vi "_Main_05_by_runs.vi"() -> ()   [LabVIEW 2017]
panel:
  out "Log N":u32
  out "Temp, C":dbl
  out "Temp_sp, C":dbl
  out "Temp_gsp, C":dbl
  in  "Start":bool
  in  "SendPeriod, ms":dbl=20.0 min=10.0 max=10000.0
  in  "Graph every, cycle":dbl=1.0 min=1.0 max=100.0
  out "Frame In Run Done":u32
  out "Now is Run #":u32
  out "Global Frame Done":u32
  in  "Frames In Run":u32=180
  in  "Exposition, s":dbl=5.0 min=0.1 max=10.0
  out "Last TrigTimer, s":dbl format="%#.3g"
  in  "LOG file":path=path "F:/_OneDrive/YandexDisk/YandexDisk/Компьютер MAINHOMEPC/OneDrive - Personal/_RF/_Проекты/Термоконтроллер/programming/LabView Side/Null_Log.txt"
  out "Flags":T1
  out "Red LED":bool
  out "Green LED":bool
  in  "Speed, K/min":dbl=5.0 min=0.1 max=10.0
  in  "Target, K":dbl=295.0 min=195.0 max=395.0
  in  "Ramp":bool
  out "Power LOG":cluster{dbl[], dbl[]}(graph)
  in  "Set temp":dbl=195.0 min=195.0 max=395.0
  in  "Setpoint":bool
  out "TrigTimer, s":dbl format="%#_3g"
  out "Vout, V":dbl format="%#.3g"
  out "Vin, V":dbl format="%#.4g"
  out "Temp, K":dbl
  out "Temp_sp, K":dbl
  out "Temp_gsp, K":dbl
  out "Temp LOG":cluster{dbl[], dbl[]}(graph)
  out "Bytes at Port":u32
  out "RecTry":i32
  in  "Stop Button":bool
  in  "COM port":refnum<visa-resource-name>
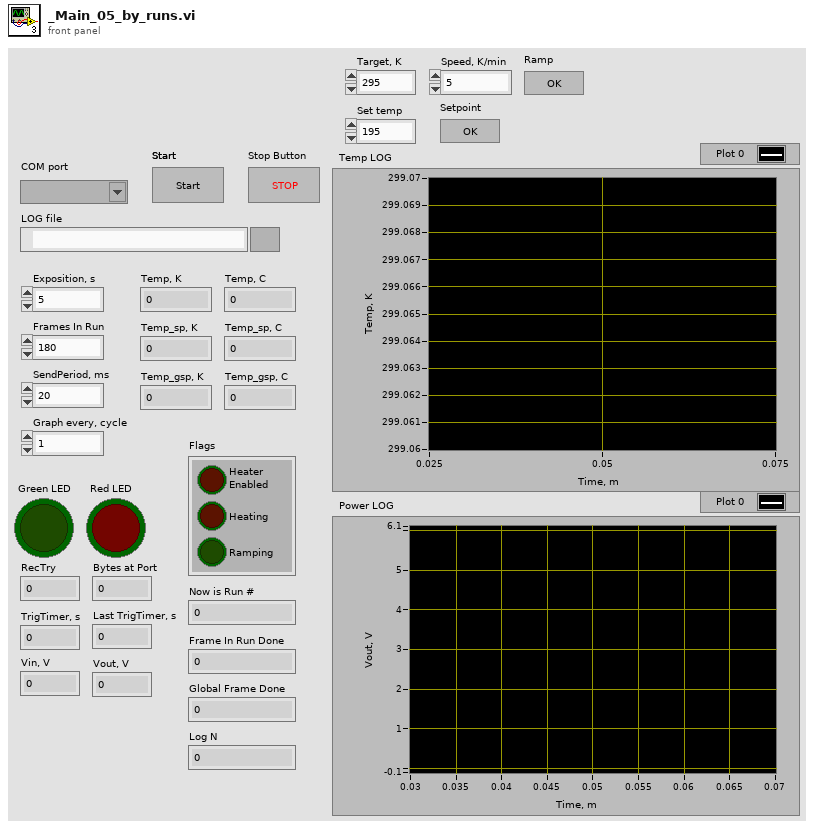
[diagram p1: front panel]
types:
  T1 = cluster{"Heater\nEnabled":bool, "Heating":bool, "Ramping":bool}
  T2 = cluster{i32, i32, u32, "Green LED":bool, "TrigTimer, s":dbl}
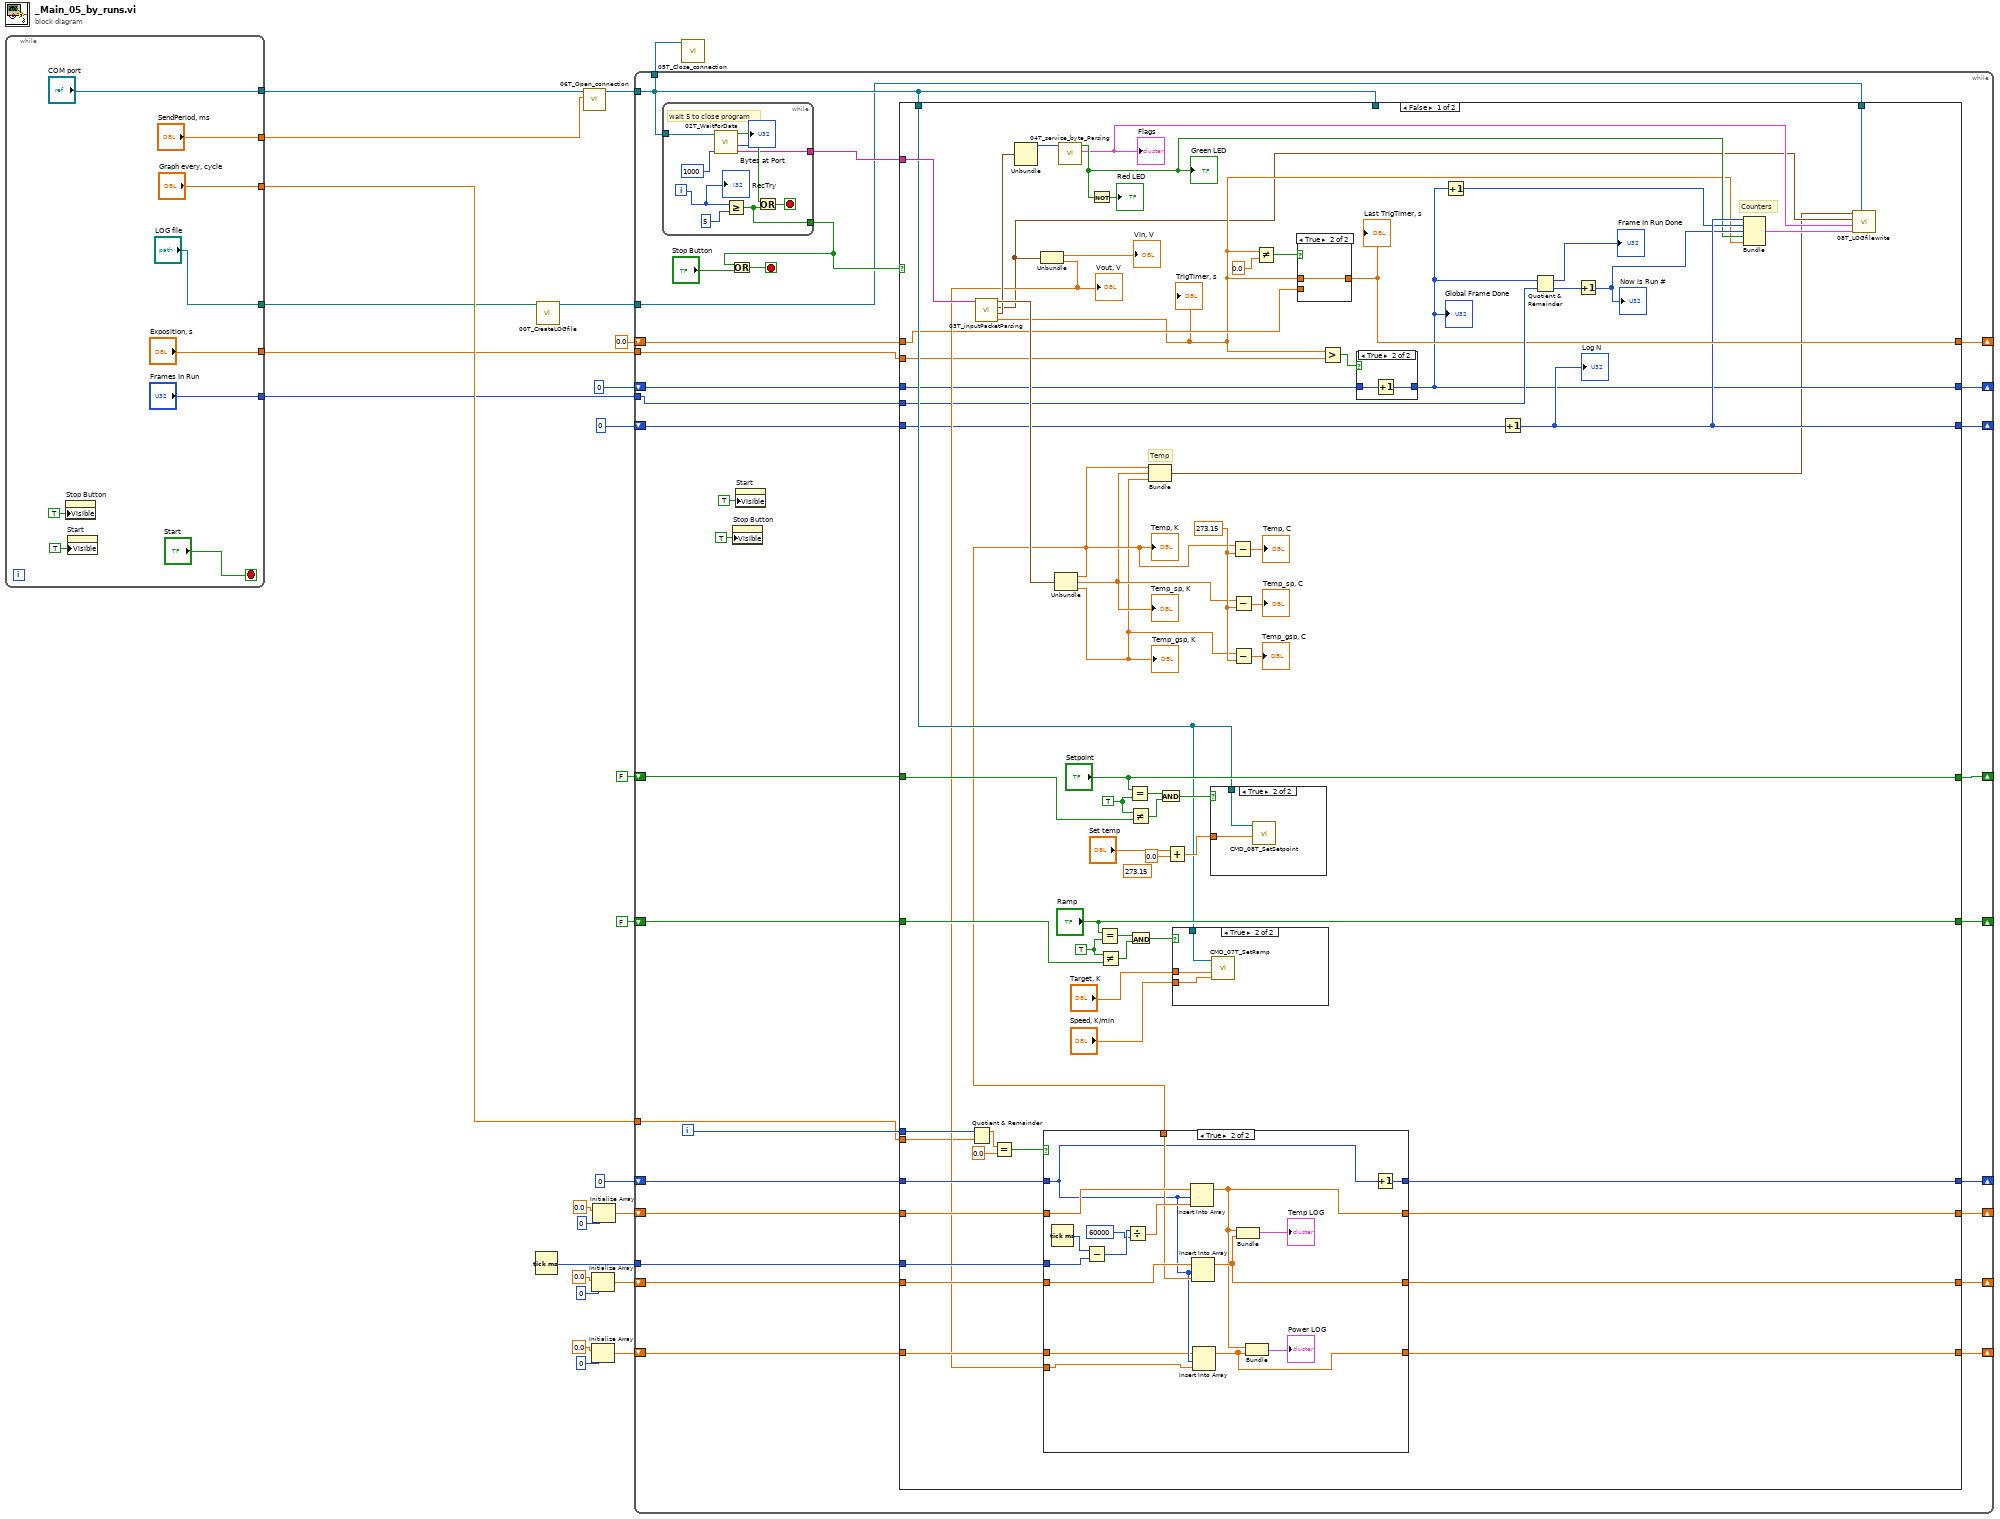
[diagram p0: block diagram]
diagram:
  n1 = while {
    tunnel: ["COM port"] -> w6
    tunnel: ["SendPeriod, ms"] -> w5
    tunnel: ["Graph every, cycle"] -> w4
    tunnel: ["LOG file"] -> w3
    tunnel: ["Frames In Run"] -> w2
    tunnel: ["Exposition, s"] -> w1
    stop <- "Start" stop-if-true
    n2 = property on="Stop Button" class="Bool"("Visible"=TRUE) -> ()  [unwired: 2 in, 2 out]
    n3 = property on="Start" class="Bool"("Visible"=TRUE) -> ()  [unwired: 2 in, 2 out]
  }
  n4 = Tick Count (ms)() -> (millisecond timer value=w21:u32)
  n5 = call "00T_CreateLOGfile.vi"("LOG file"=w3) -> ("refnum out"=w7:refnum<file>)  [unwired: 10 in]
  n6 = call "06T_Open_connection.vi"("Period, ms"=w5, "COM port"=w6) -> ("VISA"=w11:refnum<visa-resource-name>)  [unwired: 9 in]
  n7 = Initialize Array(0.0 ("element"), 0 ("dimension size")) -> (w18:dbl[])
  n8 = Initialize Array(0.0 ("element"), 0 ("dimension size")) -> (w14:dbl[])
  n9 = Initialize Array(0.0 ("element"), 0 ("dimension size")) -> (w22:dbl[])
  n10 = while {
    tunnel: w11 -> [w51]
    tunnel: [w51] -> w12
    shift-right: [w60] -> _
    shift-left: 0 -> [w61]
    tunnel: w21 -> [w58]
    shift-right: [w56] -> _
    shift-left: w22 -> [w59]
    shift-right: [w55] -> _
    shift-left: w18 -> [w57]
    shift-right: [w53] -> _
    shift-left: FALSE ("OK Button") -> [w52]
    shift-right: [w49] -> _
    shift-left: w14 -> [w50]
    shift-right: [w48] -> _
    shift-left: FALSE ("Ramp") -> [w47]
    shift-right: [w46] -> _
    shift-left: 0.0 ("TrigTimer, s") -> [w45]
    shift-right: [w43] -> _
    shift-left: 0 -> [w44]
    shift-right: [w41] -> _
    shift-left: 0 -> [w42]
    tunnel: w7 -> [w40]
    tunnel: w4 -> [w39]
    tunnel: w2 -> [w38]
    tunnel: w1 -> [w37]
    i -> [w62]
    stop <- w65 stop-if-true
    n11 = while {
      tunnel: w51 -> [w174]
      tunnel: [w177] -> w64
      tunnel: [w178] -> w63
      i -> [w176]
      stop <- w180 stop-if-true
      # "wait 5 to close program"
      n12 = call "02T_WaitForData.vi"("WaitTimeoutMS"=u32 1000, "VISA"=w174) -> ("Buffer"=w178:string, "Bytes at Port"=→"Bytes at Port":u32, "Data Recived"=w179:bool)  [unwired: 7 in]
      n13 = Greater Or Equal?(x=w176, y=5) -> (x >= y?=w177:bool)
      n14 = Or(x=w179, y=w177) -> (x .or. y?=w180:bool)
      "RecTry" <- w176
    }
    n15 = Or(x=w64, y="Stop Button") -> (x .or. y?=w65:bool)
    n16 = property on="Stop Button" class="Bool"("Visible"=TRUE) -> ()  [unwired: 2 in, 2 out]
    n17 = property on="Start" class="Bool"("Visible"=TRUE) -> ()  [unwired: 2 in, 2 out]
    n18 = case shown="False" w64 {
      tunnel: w63 -> [w125 _]
      tunnel: w62 -> [w131 _]
      tunnel: w51 -> [_ _]
      tunnel: w61 -> [w129 w173]
      tunnel: [w128 w173] -> w60
      tunnel: w59 -> [w121 w172]
      tunnel: w58 -> [w127 _]
      tunnel: w57 -> [w120 w171]
      tunnel: [w126 w172] -> w56
      tunnel: [w113 w171] -> w55
      tunnel: ["Setpoint" w170] -> w53
      tunnel: w52 -> [w117 w170]
      tunnel: w51 -> [w101 _]
      tunnel: w50 -> [w109 w169]
      tunnel: [w108 w169] -> w49
      tunnel: ["Ramp" w168] -> w48
      tunnel: w47 -> [w103 w168]
      tunnel: [w85 w167] -> w46
      tunnel: w45 -> [w93 w167]
      tunnel: w37 -> [w86 _]
      tunnel: w44 -> [w91 w166]
      tunnel: [w78 w166] -> w43
      tunnel: w38 -> [w90 _]
      tunnel: w39 -> [w87 _]
      tunnel: w42 -> [w80 w165]
      tunnel: [w79 w165] -> w41
      tunnel: w40 -> [w66 _]
      frame False {
        w81 = 273.15
        w104 = TRUE ("y")
        (unwired) 273.15 ("y")
        w116 = TRUE ("x")
        # "Counters"
        # "Temp"
        n19 = Quotient & Remainder(x=w131, y=w87) -> (x-y*floor(x/y)=w133:dbl)  [unwired: 1 out]
        n20 = call "03T_inputPacketParsing.vi"("string"=w125) -> ("TrigTimer, s"=w74:dbl, "Service"=w123:cluster{i32, i32, i32, i32}, "Voltage"=w68:cluster{dbl, dbl}, "Temp"=w124:cluster{dbl, dbl, dbl})  [unwired: 7 in]
        "TrigTimer, s" <- w74
        n21 = Equal?(x=w133, y=0.0) -> (x = y?=w130:bool)
        n22 = Unbundle(w123) -> (w98:i32)  [unwired: 3 out]
        n23 = Unbundle(w68) -> (→"Vin, V":dbl, w96:dbl)
        "Vout, V" <- w96
        n24 = Unbundle(w124) -> (w73:dbl, w72:dbl, w71:dbl)
        "Temp_gsp, K" <- w71
        "Temp_sp, K" <- w72
        "Temp, K" <- w73
        n25 = case shown="True" w130 {
          tunnel: w129 -> [w147 w153]
          tunnel: [w147 w160] -> w128
          tunnel: w121 -> [w145 w158]
          tunnel: w127 -> [_ w163]
          tunnel: w120 -> [w146 w157]
          tunnel: [w146 w155] -> w113
          tunnel: [w145 w151] -> w126
          tunnel: w73 -> [_ w154]
          tunnel: w109 -> [w144 w152]
          tunnel: [w144 w149] -> w108
          tunnel: w96 -> [_ w148]
          frame False {
          }
          frame True {
            n26 = Tick Count (ms)() -> (millisecond timer value=w164:u32)
            n27 = Subtract(x=w164, y=w163) -> (x-y=w162:u32)
            n28 = Divide(x=w162, y=u32 60000) -> (x/y=w159:dbl)
            n29 = Insert Into Array(array=w158, index=w153, new element=w159) -> (w151:dbl[])
            n30 = Insert Into Array(array=w157, index=w153, new element=w154) -> (w155:dbl[])
            n31 = Insert Into Array(array=w152, index=w153, new element=w148) -> (w149:dbl[])
            n32 = Bundle(w151, w155) -> (→"Temp LOG":cluster{dbl[], dbl[]})  [unwired: 1 in]
            n33 = Bundle(w151, w149) -> (→"Power LOG":cluster{dbl[], dbl[]})  [unwired: 1 in]
            n34 = Increment(x=w153) -> (x+1=w160:i32)
          }
        }
        n35 = call "04T_service_byte_Parsing.vi"("Service Byte"=w98) -> ("Flags"=w69:T1, "Green LED"=w75:bool)  [unwired: 9 in]
        "Green LED" <- w75
        "Flags" <- w69
        n36 = Not(x=w75) -> (.not. x?=→"Red LED":bool)
        n37 = Equal?(x="Ramp", y=w104) -> (x = y?=w107:bool)
        n38 = Not Equal?(x=w104, y=w103) -> (x != y?=w106:bool)
        n39 = Equal?(x="Setpoint", y=w116) -> (x = y?=w119:bool)
        n40 = Not Equal?(x=w116, y=w117) -> (x != y?=w115:bool)
        n41 = And(x=w107, y=w106) -> (x .and. y?=w102:bool)
        n42 = Bundle(w73, w72, w71) -> (w67:cluster{dbl, dbl, dbl})  [unwired: 1 in]
        n43 = And(x=w119, y=w115) -> (x .and. y?=w114:bool)
        n44 = Add(x="Set temp", y=0.0) -> (x+y=w112:dbl)
        n45 = case shown="True" w102 {
          tunnel: w101 -> [_ w141]
          tunnel: "Target, K" -> [_ w140]
          tunnel: "Speed, K/min" -> [_ w139]
          frame False {
          }
          frame True {
            n46 = call "CMD_07T_SetRamp.vi"("Ramp speed, K/min"=w139, "Target, K"=w140, "VISA resource name"=w141) -> ()  [unwired: 7 in, 2 out]
          }
        }
        n47 = case shown="True" w114 {
          tunnel: w112 -> [_ w143]
          tunnel: w101 -> [_ w142]
          frame False {
          }
          frame True {
            n48 = call "CMD_08T_SetSetpoint.vi"("Setpoint, K"=w143, "VISA resource name"=w142) -> ()  [unwired: 9 in, 1 out]
          }
        }
        n49 = Subtract(x=w73, y=w81) -> (x-y=→"Temp, C":dbl)
        n50 = Subtract(x=w72, y=w81) -> (x-y=→"Temp_sp, C":dbl)
        n51 = Subtract(x=w71, y=w81) -> (x-y=→"Temp_gsp, C":dbl)
        n52 = Not Equal?(x=w74, y=0.0) -> (x != y?=w94:bool)
        n53 = case shown="True" w94 {
          tunnel: w74 -> [_ w138]
          tunnel: w93 -> [w137 _]
          tunnel: [w137 w138] -> w85
          frame False {
          }
          frame True {
          }
        }
        "Last TrigTimer, s" <- w85
        n54 = Greater?(x=w74, y=w86) -> (0:w92:bool)
        n55 = case shown="True" w92 {
          tunnel: w91 -> [w134 w136]
          tunnel: [w134 w135] -> w78
          frame False {
          }
          frame True {
            n56 = Increment(x=w136) -> (x+1=w135:i32)
          }
        }
        "Global Frame Done" <- w78
        n57 = Increment(x=w78) -> (x+1=w77:i32)
        n58 = Increment(x=w80) -> (x+1=w79:i32)
        "Log N" <- w79
        n59 = Quotient & Remainder(x=w78, y=w90) -> (x-y*floor(x/y)=→"Frame In Run Done":u32, floor(x/y)=w89:u32)
        n60 = Increment(x=w89) -> (x+1=w76:u32)
        "Now is Run #" <- w76
        n61 = Bundle(w79, w77, w76, "Green LED"=w75, "TrigTimer, s"=w74) -> (w70:T2)  [unwired: 1 in]
        n62 = call "08T_LOGfilewrite.vi"("refnum out"=w66, "Counters"=w70, "Flags"=w69, "Voltage"=w68, "Temp"=w67) -> ()  [unwired: 7 in]
      }
      frame True {
      }
    }
  }
  n63 = call "05T_Close_connection.vi"("VISA"=w12) -> ()  [unwired: 11 in]
